vi "Write Container ID.vi"(8 "error in (no error)":errorcluster, 10 "Container ID":string, 11 "DataContainer in":refnum<class "DataContainer.lvclass">) -> (0 "error out":errorcluster, 3 "DataContainer out":refnum<class "DataContainer.lvclass">)   [LabVIEW 2023, in "DataContainer.lvclass"]
uses:
  DataContainer.lvclass
  DataContainer.lvclass/DataContainer.ctl
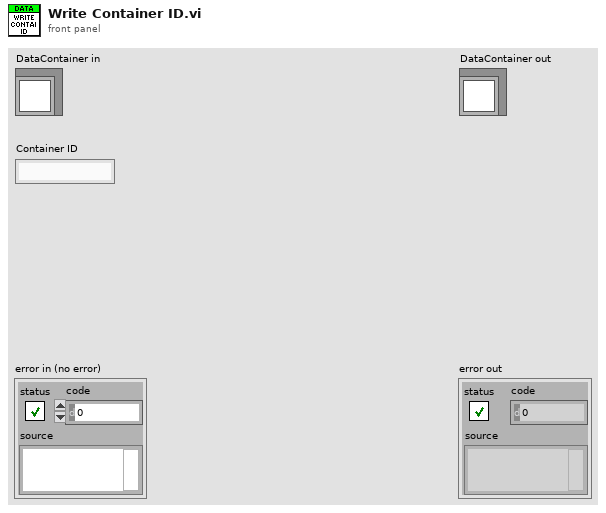
[diagram p1: front panel]
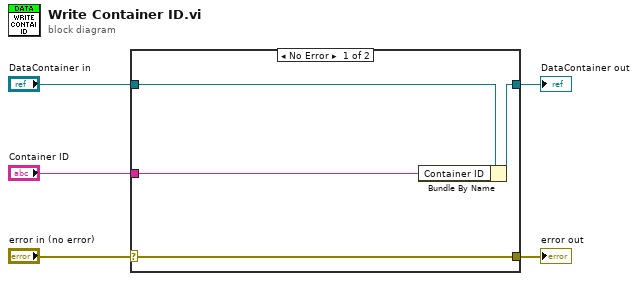
[diagram p0: block diagram]
diagram:
  n1 = case shown="No Error" "error in (no error)" {
    selector: "error in (no error)" -> [w9 w10]
    tunnel: [w9 w10] -> w4
    tunnel: [w7 w11] -> w2
    tunnel: "DataContainer in" -> [w8 w11]
    tunnel: "Container ID" -> [w6 _]
    frame No Error {
      n2 = Bundle By Name(cluster=w8, "Container ID"=w6) -> (w7:refnum<class "DataContainer.lvclass">)
    }
    frame Error {
    }
  }
  "error out" <- w4
  "DataContainer out" <- w2
